vi "Swerve Sensors RefNum Get.vi"(11 "Swerve Sensors RefNum":string) -> (3 "Swerve Sensors DevRef":T1)   [LabVIEW 2014]
uses:
  Swerve Sensors DevRef.ctl
  <vilib>/Rock Robotics/WPI/AnalogChannel/WPI_AnalogChannelDevRef.ctl
  <vilib>/Rock Robotics/SystemInterfaces/Typedef/FPGA_TypedefAnalogModule.ctl
  <vilib>/Rock Robotics/SystemInterfaces/AI/FPGA_AIChannel.ctl
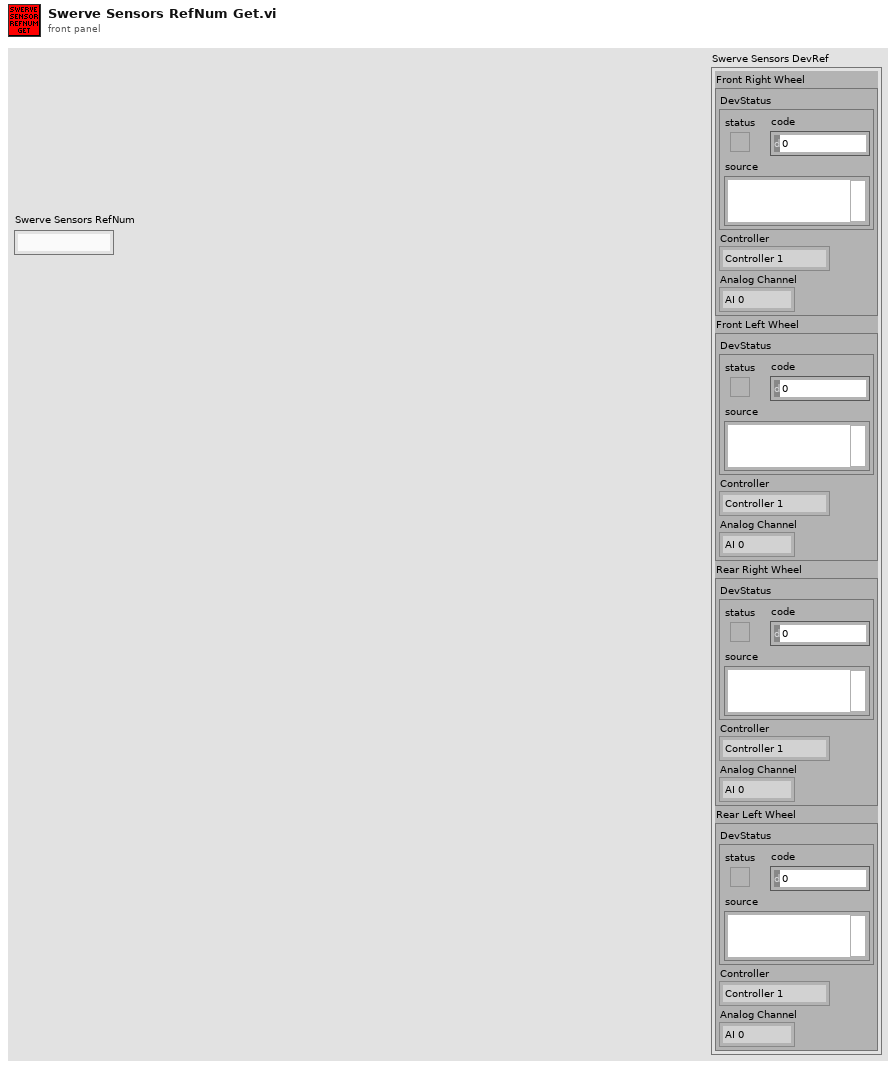
[diagram p1: front panel]
types:
  T1 = typedef "Swerve Sensors DevRef.ctl" = cluster{"Front Right Wheel":T2, "Front Left Wheel":T2, "Rear Right Wheel":T2, "Rear Left Wheel":T2}
  T2 = typedef "WPI_AnalogChannelDevRef.ctl" = cluster{"DevStatus":errorcluster, "Controller":T3, "Analog Channel":T4}
  T3 = typedef "FPGA_TypedefAnalogModule.ctl" = enum16{"Controller 1"}
  T4 = typedef "FPGA_AIChannel.ctl" = enum8{"AI 0", "AI 1", "AI 2", "AI 3", "AI MXP 0", "AI MXP 1", "AI MXP 2", "AI MXP 3", "Invalid"}
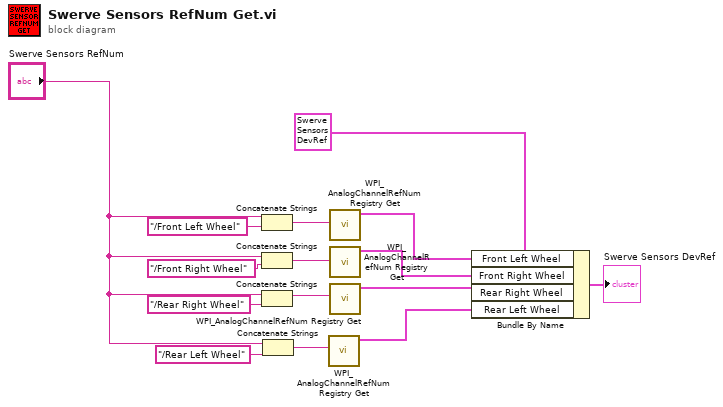
[diagram p0: block diagram]
diagram:
  n1 = Concatenate Strings("Swerve Sensors RefNum", "/Front Left Wheel" ("string")) -> (w10:string)
  n2 = Concatenate Strings("Swerve Sensors RefNum", "/Front Right Wheel" ("string")) -> (w9:string)
  n3 = Concatenate Strings("Swerve Sensors RefNum", "/Rear Right Wheel" ("string")) -> (w8:string)
  n4 = Concatenate Strings("Swerve Sensors RefNum", "/Rear Left Wheel" ("string")) -> (w7:string)
  n5 = call <vilib>:"WPI_AnalogChannelRefNum Registry Get.vi"("refnum name"=w7) -> ("AIDeviceRef"=w3:T2)  [unwired: 9 in, 1 out]
  n6 = call <vilib>:"WPI_AnalogChannelRefNum Registry Get.vi"("refnum name"=w10) -> ("AIDeviceRef"=w6:T2)  [unwired: 9 in, 1 out]
  n7 = call <vilib>:"WPI_AnalogChannelRefNum Registry Get.vi"("refnum name"=w9) -> ("AIDeviceRef"=w5:T2)  [unwired: 9 in, 1 out]
  n8 = call <vilib>:"WPI_AnalogChannelRefNum Registry Get.vi"("refnum name"=w8) -> ("AIDeviceRef"=w4:T2)  [unwired: 9 in, 1 out]
  n9 = Bundle By Name(cluster=T1 {"Front Right Wheel"={"DevStatus"={"status"=FALSE, "code"=0, "source"=""}, "Controller"=enum."Controller 1", "Analog Channel"=enum."AI 0"}, "Front Left Wheel"={"DevStatus"={"status"=FALSE, "code"=0, "source"=""}, "Controller"=enum."Controller 1", "Analog Channel"=enum."AI 0"}, "Rear Right Wheel"={"DevStatus"={"status"=FALSE, "code"=0, "source"=""}, "Controller"=enum."Controller 1", "Analog Channel"=enum."AI 0"}, "Rear Left Wheel"={"DevStatus"={"status"=FALSE, "code"=0, "source"=""}, "Controller"=enum."Controller 1", "Analog Channel"=enum."AI 0"}} ("Swerve Sensors DevRef 2"), "Front Left Wheel"=w6, "Front Right Wheel"=w5, "Rear Right Wheel"=w4, "Rear Left Wheel"=w3) -> (→"Swerve Sensors DevRef":T1)
